vi "CheckPressure.vi"(8 "error in (no error)":errorcluster, 11 "UI.lvclass":refnum<class "S1.lvclass">) -> (0 "error out":errorcluster, 3 "UI.lvclass":refnum<class "S1.lvclass">)   [LabVIEW 2018, in "S1.lvclass"]
uses:
  S1.lvclass
  S1.lvclass/S1.ctl
  Public Controls/ReportHeader.ctl
  Controller/GUI.lvclass
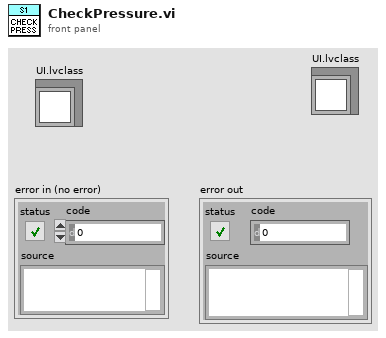
[diagram p1: front panel]
types:
  T1 = typedef "S1.lvclass/ReportHeader.ctl" = string
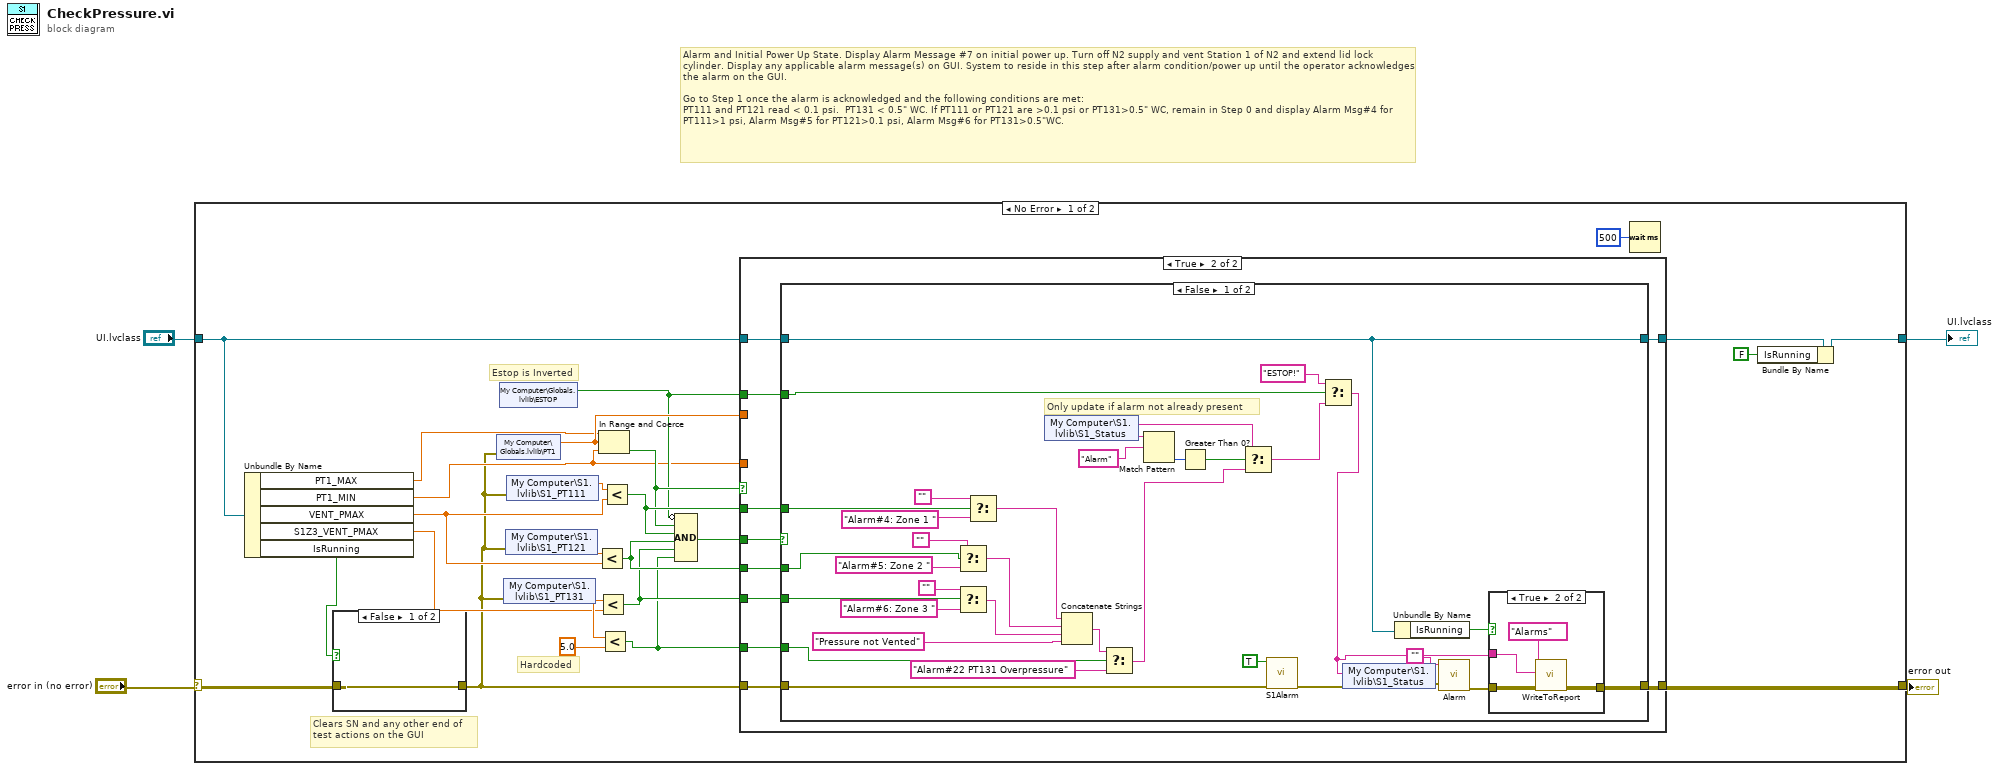
[diagram p0: block diagram]
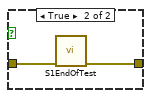
[diagram p2: hidden frame]
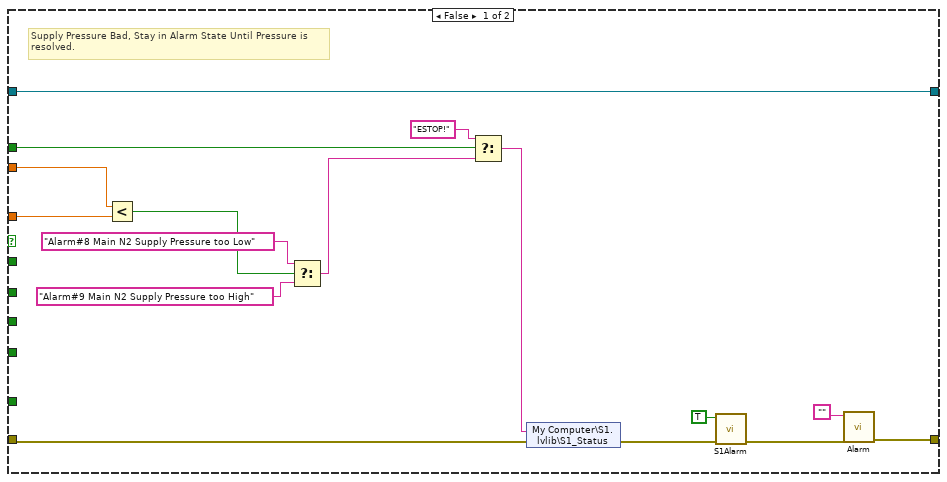
[diagram p3: hidden frame]
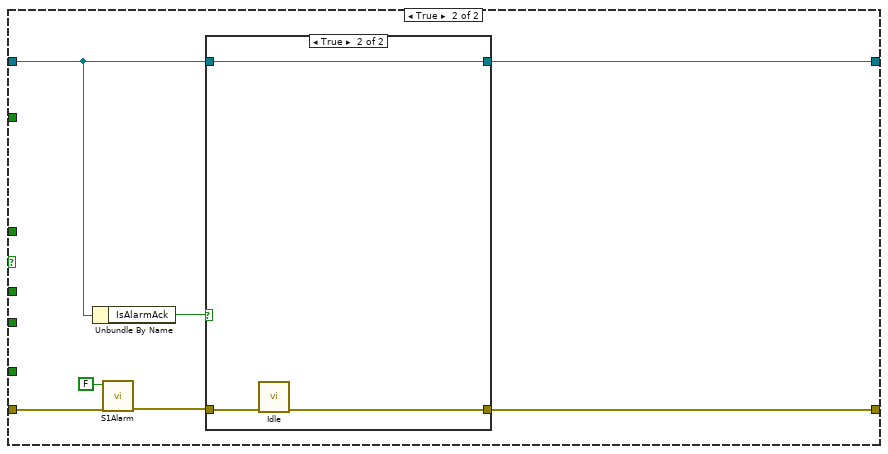
[diagram p5: hidden frame]
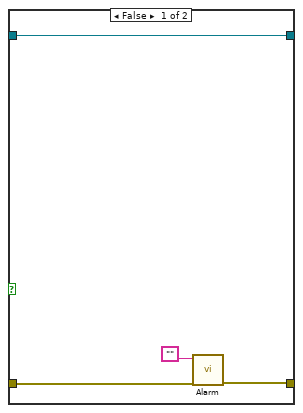
[diagram p6: hidden frame]
diagram:
  # "Alarm and Initial Power Up State. Display Alarm Message #7 on initial power up. Turn off N2 supply and vent Station 1 of N2 and extend lid lock cylinder. Display any applicable alarm message(s) on GUI. System to reside in this step after alarm condition/power up until the operator acknowledges the alarm on the GUI. \n\nGo to Step 1 once the alarm is acknowledged and the following conditions are met:\nPT111 and PT121 read < 0.1 psi.  PT131 < 0.5\" WC. If PT111 or PT121 are >0.1 psi or PT131>0.5\" WC, remain in Step 0 and display Alarm Msg#4 for PT111>1 psi, Alarm Msg#5 for PT121>0.1 psi, Alarm Msg#6 for PT131>0.5\"WC."
  n1 = case shown="No Error" "error in (no error)" {
    selector: "error in (no error)" -> [w6 w113]
    tunnel: [w26 w113] -> w3
    tunnel: "UI.lvclass" -> [w14 w112]
    tunnel: [w9 w112] -> w1
    frame No Error {
      # "Clears SN and any other end of\ntest actions on the GUI"
      # "Hardcoded"
      # "Estop is Inverted"
      n2 = Unbundle By Name(w14) -> ("PT1_MAX"=w11:dbl, "PT1_MIN"=w10:dbl, "VENT_PMAX"=w13:dbl, "S1Z3_VENT_PMAX"=w12:dbl, "IsRunning"=w7:bool)
      n3 = case shown="False" w7 {
        tunnel: w6 -> [w30 w32]
        tunnel: [w30 w31] -> w5
        frame False {
        }
        frame True {
          n4 = call "S1EndOfTest.vi"("error in"=w32) -> ("error out"=w31:errorcluster)  [unwired: 10 in]
        }
      }
      n5 = shared-variable "My Computer\\Globals.lvlib\\PT1"(error in=w5) -> (w21:dbl)  [unwired: 1 out]
      n6 = shared-variable "My Computer\\Globals.lvlib\\ESTOP"() -> (w16:bool)  [unwired: 1 in, 1 out]
      n7 = shared-variable "My Computer\\S1.lvlib\\S1_PT131"(error in=w5) -> (w19:dbl)  [unwired: 1 out]
      n8 = shared-variable "My Computer\\S1.lvlib\\S1_PT121"(error in=w5) -> (w28:dbl)  [unwired: 1 out]
      n9 = shared-variable "My Computer\\S1.lvlib\\S1_PT111"(error in=w5) -> (w29:dbl)  [unwired: 1 out]
      n10 = Less?(x=w28, y=w13) -> (x < y?=w24:bool)
      n11 = Less?(x=w19, y=w12) -> (x < y?=w23:bool)
      n12 = In Range and Coerce(upper limit=w11, x=w21, lower limit=w10) -> (In Range?=w22:bool)  [unwired: 1 out]
      n13 = Less?(x=w19, y=5.0) -> (x < y?=w17:bool)
      n14 = Less?(x=w29, y=w13) -> (x < y?=w25:bool)
      n15 = Compound Arithmetic op=AND(invert w16, w22, w25, w24, w23, w17) -> (w27:bool)
      n16 = case shown="True" w22 {
        tunnel: w27 -> [_ w58]
        tunnel: [w44 w57] -> w26
        tunnel: w25 -> [_ w56]
        tunnel: w24 -> [_ w55]
        tunnel: w23 -> [_ w54]
        tunnel: w5 -> [w45 w53]
        tunnel: w21 -> [w48 _]
        tunnel: w10 -> [w42 _]
        tunnel: w17 -> [_ w52]
        tunnel: w16 -> [w36 w51]
        tunnel: w14 -> [w41 w50]
        tunnel: [w41 w49] -> w15
        frame False {
          # "Supply Pressure Bad, Stay in Alarm State Until Pressure is\nresolved."
          n17 = Less?(x=w48, y=w42) -> (x < y?=w47:bool)
          n18 = Select(t="Alarm#8 Main N2 Supply Pressure too Low" ("Status"), s=w47, f="Alarm#9 Main N2 Supply Pressure too High" ("Status")) -> (s? t:f=w35:string)
          n19 = Select(t="ESTOP!" ("Status"), s=w36, f=w35) -> (s? t:f=w34:string)
          n20 = shared-variable "My Computer\\S1.lvlib\\S1_Status"(w34, error in=w45) -> (error out=w39:errorcluster)
          n21 = call "S1Alarm.vi"("error in"=w39, "HasAlarm"=TRUE) -> ("error out"=w38:errorcluster)  [unwired: 9 in]
          n22 = call "Alarm.vi"("error in"=w38, "Alarm"="") -> ("error out"=w44:errorcluster)  [unwired: 9 in]
        }
        frame True {
          n23 = case shown="False" w58 {
            tunnel: w53 -> [w69 w99]
            tunnel: [w75 w104] -> w57
            tunnel: w56 -> [w90 _]
            tunnel: w55 -> [w86 _]
            tunnel: w54 -> [w84 _]
            tunnel: w52 -> [w79 _]
            tunnel: w51 -> [w62 _]
            tunnel: w50 -> [w71 w102]
            tunnel: [w71 w101] -> w49
            frame False {
              # "Only update if alarm not already present"
              n24 = Select(t="", s=w86, f="Alarm#5: Zone 2 " ("Status")) -> (s? t:f=w81:string)
              n25 = Select(t="", s=w84, f="Alarm#6: Zone 3 " ("Status")) -> (s? t:f=w80:string)
              n26 = Select(t="", s=w90, f="Alarm#4: Zone 1 " ("Status")) -> (s? t:f=w82:string)
              n27 = shared-variable "My Computer\\S1.lvlib\\S1_Status"() -> (w64:string)  [unwired: 1 in, 1 out]
              n28 = Concatenate Strings(w82, w81, w80, "Pressure not Vented" ("Status")) -> (w78:string)
              n29 = Select(t=w78, s=w79, f="Alarm#22 PT131 Overpressure") -> (s? t:f=w63:string)
              n30 = Match Pattern(string=w64, regular expression="Alarm") -> (offset past match=w66:i32)  [unwired: 1 in, 3 out]
              n31 = Greater Than 0?(x=w66) -> (x > 0?=w65:bool)
              n32 = Select(t=w64, s=w65, f=w63) -> (s? t:f=w61:string)
              n33 = call "S1Alarm.vi"("error in"=w69, "HasAlarm"=TRUE) -> ("error out"=w68:errorcluster)  [unwired: 9 in]
              n34 = Select(t="ESTOP!" ("Status"), s=w62, f=w61) -> (s? t:f=w60:string)
              n35 = shared-variable "My Computer\\S1.lvlib\\S1_Status"(w60, error in=w68) -> (error out=w92:errorcluster)
              n36 = Unbundle By Name(w71) -> ("IsRunning"=w72:bool)
              n37 = call "Alarm.vi"("error in"=w92, "Alarm"="") -> ("error out"=w76:errorcluster)  [unwired: 9 in]
              n38 = case shown="True" w72 {
                tunnel: w76 -> [w93 w97]
                tunnel: [w93 w96] -> w75
                tunnel: w60 -> [_ w94]
                frame False {
                }
                frame True {
                  n39 = call "WriteToReport.vi"("error in"=w97, "Value"=w94, "Header"=T1 "Alarms") -> ("error out"=w96:errorcluster)  [unwired: 8 in]
                }
              }
            }
            frame True {
              n40 = Unbundle By Name(w102) -> ("IsAlarmAck"=w103:bool)
              n41 = call "S1Alarm.vi"("error in"=w99, "HasAlarm"=FALSE) -> ("error out"=w98:errorcluster)  [unwired: 9 in]
              n42 = case shown="True" w103 {
                tunnel: w98 -> [w106 w111]
                tunnel: [w108 w110] -> w104
                tunnel: w102 -> [w107 w109]
                tunnel: [w107 w109] -> w101
                frame False {
                  n43 = call "Alarm.vi"("error in"=w106, "Alarm"="") -> ("error out"=w108:errorcluster)  [unwired: 9 in]
                }
                frame True {
                  n44 = call "Idle.vi"("error in"=w111) -> ("error out"=w110:errorcluster)  [unwired: 10 in]
                }
              }
            }
          }
        }
      }
      n45 = Wait (ms)(milliseconds to wait=u32 500) -> ()  [unwired: 1 out]
      n46 = Bundle By Name(cluster=w15, "IsRunning"=FALSE) -> (w9:refnum<class "S1.lvclass">)
    }
    frame Error {
    }
  }
  "error out" <- w3
  "UI.lvclass" <- w1
